vi "Get TablePart.vi"(7 "Sheet Name in":string, 8 "error in":errorcluster, 10 "TableDefinitionPart in":refnum<k24>, 11 "SpreadsheetDoc in":refnum<k24>) -> (0 "error out":errorcluster, 1 "TablePart":refnum<k24>, 2 "TableDefinitionPart out":refnum<k24>, 3 "SpreadsheetDoc out":refnum<k24>, 5 "Sheet Name out":string)   [LabVIEW 2019, in "Open Xml.lvlib"]
uses:
  Open Xml.lvlib
  D:/git/Open-Xml-LabVIEW/Source/DocumentFormat.OpenXml.dll
  DocumentFormat.OpenXml.dll
  D:/git/Open-Xml-LabVIEW/Source/DocumentFormat.OpenXml.Framework.dll
  DocumentFormat.OpenXml.Framework.dll
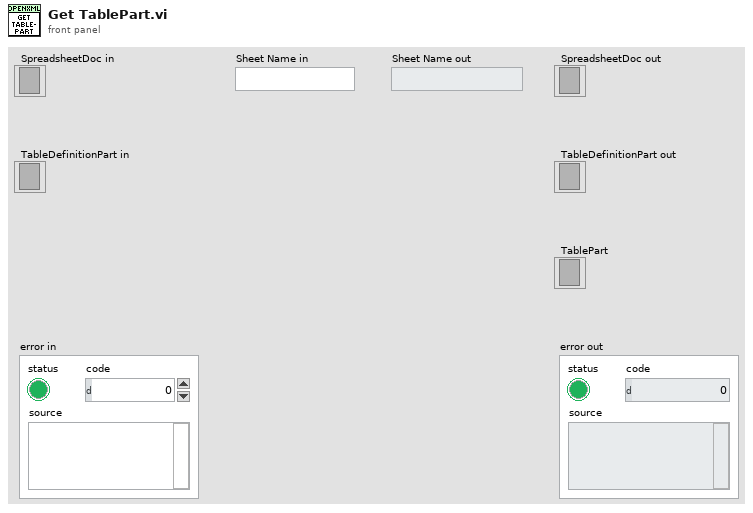
[diagram p1: front panel]
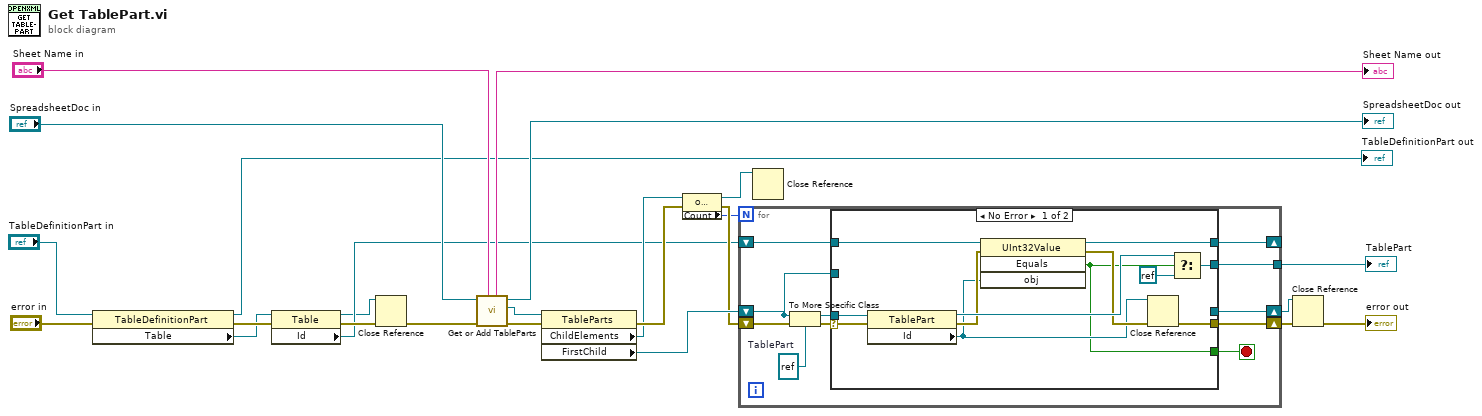
[diagram p0: block diagram]
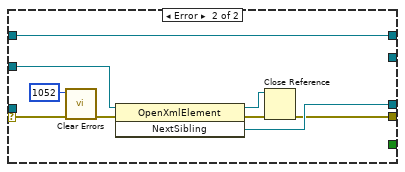
[diagram p2: hidden frame]
diagram:
  n1 = property class="TableDefinitionPart"(reference="TableDefinitionPart in", error in="error in") -> (reference out=→"TableDefinitionPart out":refnum<k24>, error out=w8:errorcluster, "Table"=w5:refnum<k24>)
  n2 = property class="Table"(reference=w5, error in=w8) -> (reference out=w1:refnum<k24>, error out=w6:errorcluster, "Id"=w3:refnum<k24>)
  n3 = Close Reference(reference=w1, error in (no error)=w6) -> (error out=w2:errorcluster)
  n4 = call "Get or Add TableParts.vi"("Sheet Name"="Sheet Name in", "error in"=w2, "SpreadsheetDoc in"="SpreadsheetDoc in") -> ("error out"=w14:errorcluster, "TableParts"=w15:refnum<k24>, "SpreadsheetDoc out"=→"SpreadsheetDoc out":refnum<k24>, "Sheet Name"=→"Sheet Name out":string)  [unwired: 5 in]
  n5 = property class="TableParts"(reference=w15, error in=w14) -> (error out=w20:errorcluster, "ChildElements"=w17:refnum<k24>, "FirstChild"=w22:refnum<k24>)  [unwired: 1 out]
  n6 = property class="OpenXmlElementList"(reference=w17, error in=w20) -> (reference out=w19:refnum<k24>, error out=w21:errorcluster, "Count"=w18:i32)
  n7 = for {
    N: w18 -> [_]
    shift-right: [w33] -> w16
    shift-left: w21 -> [w36]
    shift-right: [w30] -> w24
    shift-left: w22 -> [w31]
    tunnel: [w29] -> w25
    shift-right: [w26] -> _
    shift-left: w3 -> [w27]
    stop <- w28 stop-if-true
    w34 = refnum<k24> refnum  # TablePart
    n8 = To More Specific Class(target class=w34, reference=w31, error in=w36) -> (specific class reference=w32:refnum<k24>, error out=w35:errorcluster)
    n9 = case shown="No Error" w35 {
      selector: w35 -> [w48 w57]
      tunnel: [w41 w51] -> w33
      tunnel: w32 -> [w47 _]
      tunnel: w31 -> [_ w53]
      tunnel: [_ w52] -> w30
      tunnel: [w39 _] -> w29
      tunnel: [w38 _] -> w28
      tunnel: w27 -> [w45 w49]
      tunnel: [w44 w49] -> w26
      frame No Error {
        n10 = property class="TablePart"(reference=w47, error in=w48) -> (reference out=w46:refnum<k24>, error out=w43:errorcluster, "Id"=w40:refnum<k24>)
        n11 = invoke class="UInt32Value" method="Equals"(reference=w45, error in=w43, "obj"=w40) -> (reference out=w44:refnum<k24>, error out=w42:errorcluster, "Equals"=w38:bool)  [unwired: 1 in, 1 out]
        n12 = Close Reference(reference=w40, error in (no error)=w42) -> (error out=w41:errorcluster)
        n13 = Select(t=w46, s=w38, f=refnum<k0> refnum) -> (s? t:f=w39:refnum<k24>)
      }
      frame Error {
        n14 = call <vilib>:"Clear Errors.vi"("error in (no error)"=w57, "specific error code to clear (0: all)"=1052) -> ("error out"=w56:errorcluster)  [unwired: 4 in, 1 out]
        n15 = invoke class="OpenXmlElement" method="NextSibling"(reference=w53, error in=w56) -> (reference out=w50:refnum<k24>, error out=w54:errorcluster, "NextSibling"=w52:refnum<k24>)  [unwired: 1 in]
        n16 = Close Reference(reference=w50, error in (no error)=w54) -> (error out=w51:errorcluster)
      }
    }
  }
  "TablePart" <- w25
  n17 = Close Reference(reference=w19) -> ()  [unwired: 1 in, 1 out]
  n18 = Close Reference(reference=w24, error in (no error)=w16) -> (error out=→"error out":errorcluster)
